vi "Wait.vi"(0 "object in":refnum<class "Application.lvclass">, 2 "Wait (s)":dbl, 5 "error in (no error)":errorcluster) -> (14 "object out":refnum<class "Application.lvclass">, 19 "error out":errorcluster)   [LabVIEW 2019, in "Application.lvclass"]
uses:
  Application.lvclass
panel:
  out "Time has Elapsed":bool
  out "Elapsed Time (s)":dbl
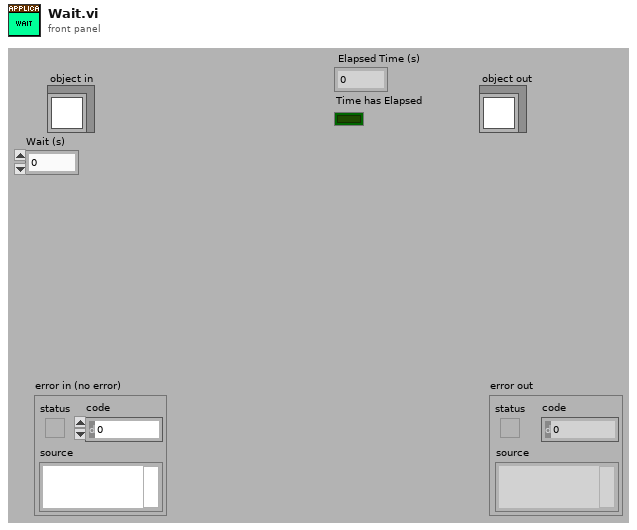
[diagram p1: front panel]
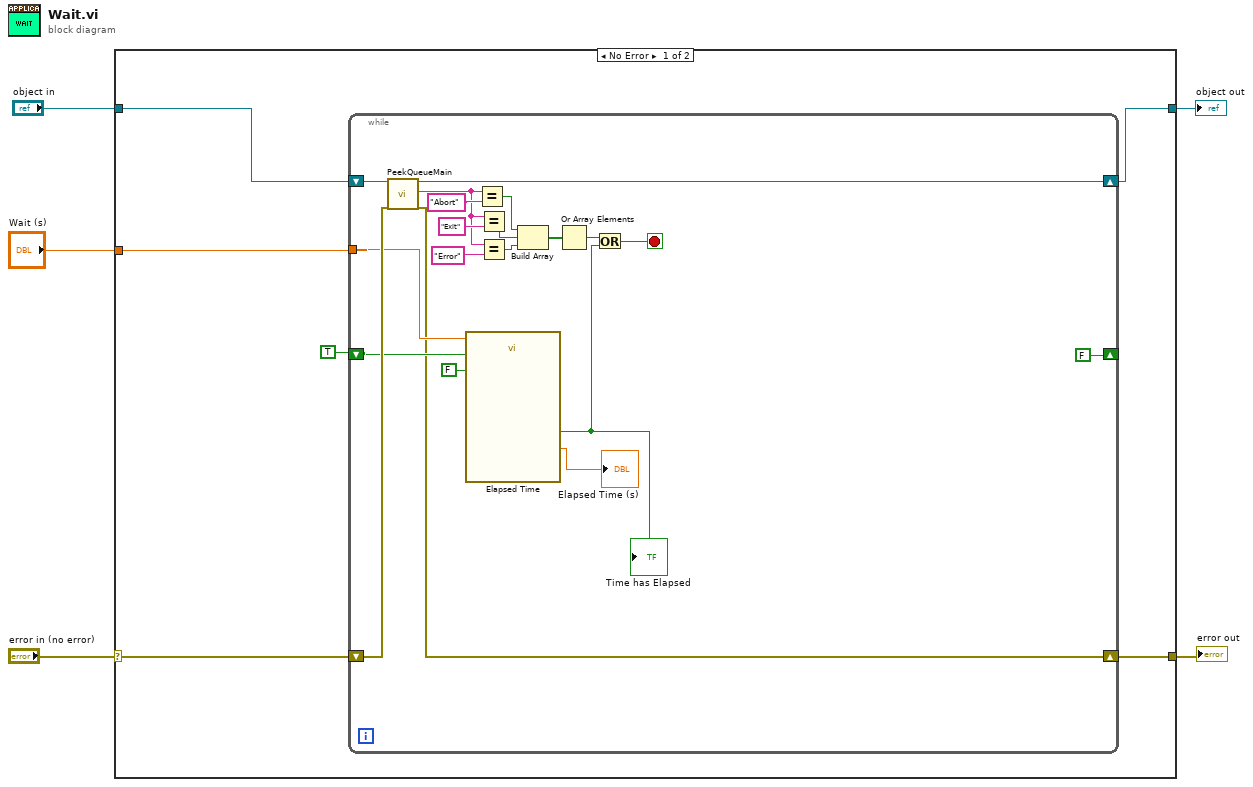
[diagram p0: block diagram]
diagram:
  n1 = case shown="No Error" "error in (no error)" {
    selector: "error in (no error)" -> [w11 w33]
    tunnel: [w10 w33] -> w4
    tunnel: [w7 w32] -> w2
    tunnel: "object in" -> [w6 w32]
    tunnel: "Wait (s)" -> [w9 _]
    frame No Error {
      n2 = while {
        shift-right: [w30] -> w7
        shift-left: w6 -> [w31]
        tunnel: w9 -> [w17]
        shift-right: [FALSE] -> _
        shift-left: TRUE -> [w18]
        shift-right: [w14] -> w10
        shift-left: w11 -> [w19]
        stop <- w20 stop-if-true
        n3 = call-dynamic "PeekQueueMain.vi"("object in"=w31, "error in (no error)"=w19) -> ("object out"=w30:refnum<class "Application.lvclass">, "Message"=w22:string, "error out"=w14:errorcluster)  [unwired: 14 in, 1 out]
        n4 = call "Elapsed Time"("Time Target (s)"=w17, "Reset"=w18, "Auto Reset"=FALSE) -> ("Elapsed Time (s)"=→"Elapsed Time (s)":dbl, "Time has Elapsed"=w13:bool)  [unwired: 9 in, 6 out]
        "Time has Elapsed" <- w13
        n5 = Equal?(x=w22, y="Abort") -> (x = y?=w25:bool)
        n6 = Equal?(x=w22, y="Exit") -> (x = y?=w24:bool)
        n7 = Equal?(x=w22, y="Error") -> (x = y?=w26:bool)
        n8 = Build Array(w25, w24, w26) -> (w23:bool[])
        n9 = Or Array Elements(Boolean array=w23) -> (logical OR=w21:bool)
        n10 = Or(x=w21, y=w13) -> (x .or. y?=w20:bool)
      }
    }
    frame Error {
    }
  }
  "error out" <- w4
  "object out" <- w2
